vi "ReflexProgram2MarcoGonzalez.vi"() -> ()   [LabVIEW 2012]
panel:
  out "Reflex Time":dbl
  in  "?":bool
  out "Light":bool
  # "Marco Gonzalez\nEA 3\n03 / 10 /2017"
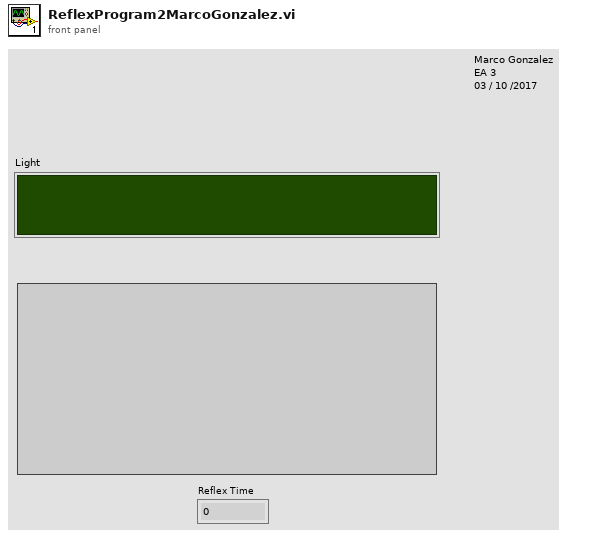
[diagram p1: front panel]
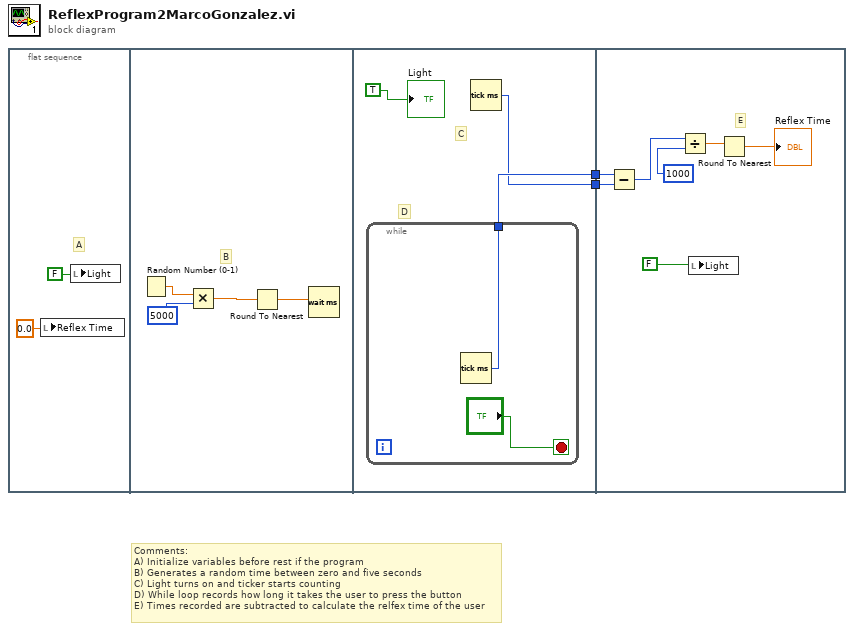
[diagram p0: block diagram]
diagram:
  # "Comments:\nA) Initialize variables before rest if the program\nB) Generates a random time between zero and five seconds\nC) Light turns on and ticker starts counting\nD) While loop records how long it takes the user to press the button\nE) Times recorded are subtracted to calculate the relfex time of the user"
  n1 = flat-sequence {
    tunnel: [w10] -> w2
    tunnel: [w9] -> w1
    tunnel: w2 -> [w17]
    tunnel: w1 -> [w16]
    frame #0 {
      # "A"
      n2 = local write "Reflex Time"(0.0 ("Reflex Time")) -> ()
      n3 = local write "Light"(FALSE) -> ()
    }
    frame #1 {
      # "B"
      n4 = Random Number (0-1)() -> (number: 0 to 1=w7:dbl)
      n5 = Multiply(x=w7, y=5000) -> (x*y=w8:dbl)
      n6 = Round To Nearest(number=w8) -> (nearest integer value=w5:dbl)
      n7 = Wait (ms)(milliseconds to wait=w5) -> ()  [unwired: 1 out]
    }
    frame #2 {
      # "D"
      # "C"
      n8 = while {
        tunnel: [w12] -> w10
        stop <- "?" stop-if-true
        n9 = Tick Count (ms)() -> (millisecond timer value=w12:u32)
      }
      n10 = Tick Count (ms)() -> (millisecond timer value=w9:u32)
      "Light" <- TRUE
    }
    frame #3 {
      # "E"
      n11 = Subtract(x=w17, y=w16) -> (x-y=w19:u32)
      n12 = Divide(x=w19, y=u32 1000) -> (x/y=w15:dbl)
      n13 = local write "Light"(FALSE) -> ()
      n14 = Round To Nearest(number=w15) -> (nearest integer value=→"Reflex Time":dbl)
    }
  }
